vi "Main.vi"(0 "PID On":bool) -> (5 "Total (V)":dbl[](array[slide]) scale=-8.0..8.0, 6 "Force (N)":T3(graph)={"M1 ref force"=20.0, "M2 ref force"=10.768311870905725, "M1 mes force"=3.690819426740976, "M2 mes force"=4.004504201458466})   [LabVIEW 2021]
uses:
  <vilib>/Platform/TimedLoop/XDataNode/timing_clust.ctl
  <vilib>/Platform/TimedLoop/XDataNode/nitl_modes.ctl
  <vilib>/Platform/TimedLoop/XDataNode/wakeup.ctl
  <vilib>/DAQmx/write.llb/DAQmx Write (Digital 1D Bool 1Chan 1Samp).vi
  <vilib>/DAQmx/write.llb/DAQmx Write (Analog 1D DBL NChan 1Samp).vi
  <vilib>/DAQmx/create/channels.llb/DAQmx Create Channel (DO-Digital Output).vi
  <vilib>/DAQmx/create/channels.llb/DAQmx Create Channel (AO-Voltage-Basic).vi
  <vilib>/DAQmx/create/channels.llb/DAQmx Create Channel (AI-Voltage-Basic).vi
  <vilib>/addons/control/pid/pid.llb/PID (DBL).vi
  <vilib>/DAQmx/miscellaneous.llb/DAQmx Fill In Error Info.vi
  <vilib>/Platform/TimedLoop/XDataNode/XDataNode.xnode
  <vilib>/Platform/TimedLoop/XDataNode/XDNodeRunTimeDep.lvlib
  <vilib>/addons/control/pid/NI_PID_pid.lvlib
panel:
  in  "Traj Start":bool
  in  "PID gains":T1={"proportional gain (Kc)"=0.15, "integral time (Ti, min)"=0.0, "derivative time (Td, min)"=0.0} {"derivative time (Td, min)" format="%.3f"; "integral time (Ti, min)" format="%.3f"; "proportional gain (Kc)" format="%.3f"}
  out "output":dbl(slide)=-9.231688129094275 scale=-40.0..40.0
  in  "Numeric":dbl=3.0
  in  "Tab Control":enum32{"PID Gain", "PIN On"}(tab)=enum."PIN On"
  in  "Gains":T2(array[cluster])=[{"proportional gain (Kc)"=0.17, "integral time (Ti, min)"=0.0, "derivative time (Td, min)"=0.0}, {"proportional gain (Kc)"=0.17, "integral time (Ti, min)"=0.0, "derivative time (Td, min)"=0.0}] {"derivative time (Td, min)" format="%.3f"; "integral time (Ti, min)" format="%.3f"; "proportional gain (Kc)" format="%.3f"}
  out "PID (V)":dbl[](array[slide])=[2.7725606974540344, 1.0] scale=-8.0..8.0
  out "Position (mm)":cluster{"Position":dbl, "ref_x (mm)":dbl}(graph)={"Position"=61.544587527295164, "ref_x (mm)"=0.0}
  in  "Loadcell":bool
  in  "Encoder Init":bool
  out "Speed (RPM)":dbl[](array[knob]) scale=-200.0..200.0
  out "time (s)":dbl=637.168
  in  "Set Point":dbl(slide)=19.690402476780186 scale=0.0..40.0
  in  "Motor Enable":bool[](array[boolean])=[FALSE, FALSE]
  in  "stop":bool
  # "FORCE"
  # "TRAJECTORY"
  # "INITIALIZE"
  # "TUNE"
  # "MONITOR"
  # "DEVEL"
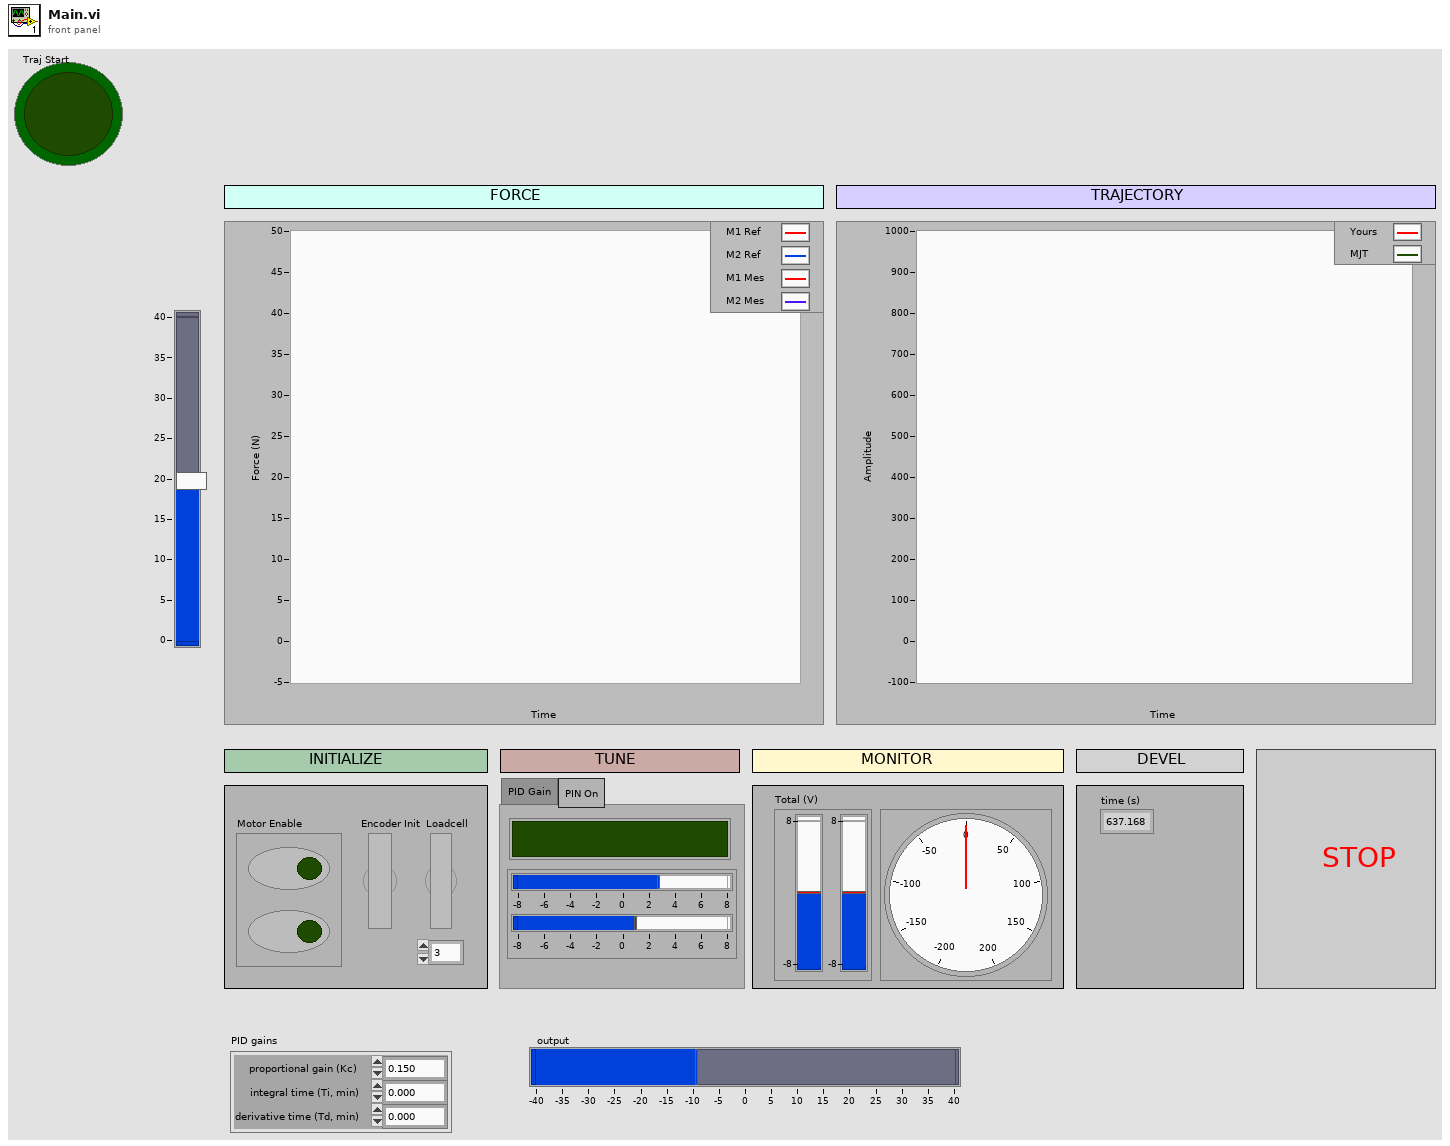
[diagram p1: front panel]
types:
  T1 = cluster{"proportional gain (Kc)":dbl, "integral time (Ti, min)":dbl, "derivative time (Td, min)":dbl}
  T2 = cluster{"proportional gain (Kc)":dbl, "integral time (Ti, min)":dbl, "derivative time (Td, min)":dbl}[]
  T3 = cluster{"M1 ref force":dbl, "M2 ref force":dbl, "M1 mes force":dbl, "M2 mes force":dbl}
  T4 = typedef "XDNodeRunTimeDep.lvlib/timing_clust.ctl" = cluster{"Expected End [f-1]":u64, "Actual End [f-1]":u64, "Finished Late? [f-1]":bool, "Expected End [i-1]":u64, "Actual End [i-1]":u64, "Finished Late? [i-1]":bool, "Expected Start [i]":u64, "Actual Start [i]":u64, "Expected Start [f]":u64, "Actual Start [f]":u64, "Source Name":string, "Structure Name":string, "Period":i64, "Deadline":i64, "Offset":i64, "Start":i64, "Priority":i32, "Timeout":i32, "Mode":T5, "Wakeup Reason":T6, "Error":errorcluster, "Source Type":string, "Secondary Source Type":string, "Global End Time":u64, "Global Start Time":u64, "Frame Duration":u64, "Iteration Duration":u64, "Assigned CPU":i32, "I/O Scan Engine Mode":u32}
  T5 = typedef "XDNodeRunTimeDep.lvlib/nitl_modes.ctl" = enum32{"No Change", "Process missed periods, maintain original phase", "Discard missed periods, maintain original phase", "Process missed periods, ignore original phase", "Discard missed periods, ignore original phase"}
  T6 = typedef "XDNodeRunTimeDep.lvlib/wakeup.ctl" = enum32{"Normal", "Aborted", "Asynchronous wakeup", "Timing source error", "Timed loop error", "Timeout"}
  T7 = cluster{"Total Time":dbl, "Total Length":dbl, "Control Freq":dbl}
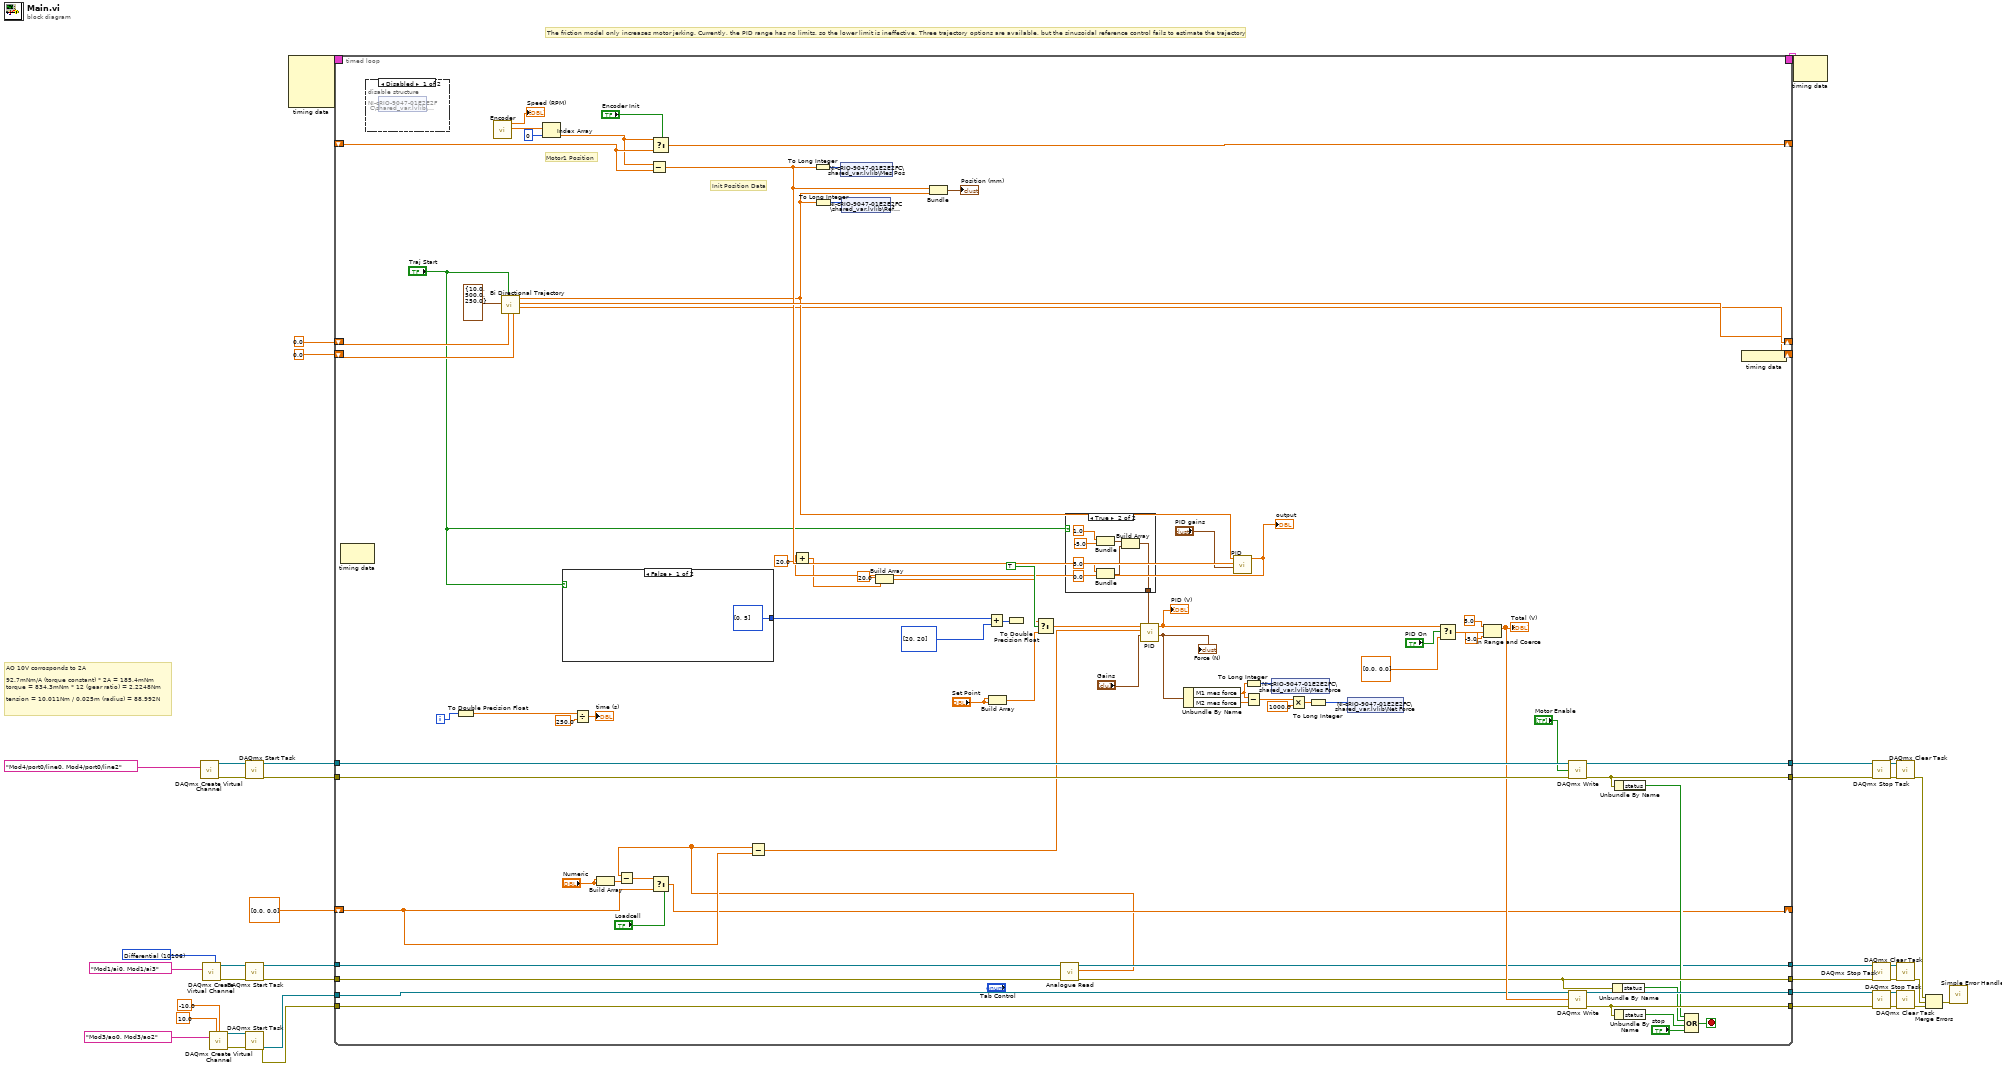
[diagram p0: block diagram]
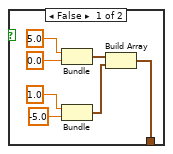
[diagram p3: hidden frame]
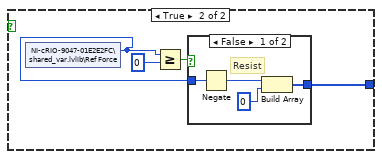
[diagram p4: hidden frame]
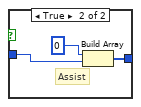
[diagram p5: hidden frame]
diagram:
  w4 = 10106 items=["Default"=-1, "RSE"=10083, "NRSE"=10078, "Differential"=10106, "Pseudodifferential"=12529] ("input terminal configuration")
  # "The friction model only increases motor jerking. Currently, the PID range has no limits, so the lower limit is ineffective. Three trajectory options are available, but the sinusoidal reference control fails to estimate the trajectory"
  # "AO 10V corrosponds to 2A\n\n92.7mNm/A (torque constant) * 2A = 185.4mNm\ntorque = 834.3mNm * 12 (gear ratio) = 2.2248Nm\n\ntension = 10.011Nm / 0.025m (radius) = 88.992N"
  n1 = call-poly <vilib>:"DAQmx Create Virtual Channel.vi"("lines"=tag "Mod4/port0/line0, Mod4/port0/line2") -> ("task out"=w31:refnum<k21>, "error out"=w30:errorcluster)  [unwired: 13 in]
  n2 = call-poly <vilib>:"DAQmx Create Virtual Channel.vi"("input terminal configuration"=w4, "physical channels"=tag "Mod1/ai0, Mod1/ai3") -> ("task out"=w21:refnum<k21>, "error out"=w22:errorcluster)  [unwired: 12 in]
  n3 = call-poly <vilib>:"DAQmx Create Virtual Channel.vi"("maximum value"=10.0 ("AO max"), "minimum value"=-10.0 ("AO min"), "physical channels"=tag "Mod3/ao0, Mod3/ao2" ("Physical Channel(s)")) -> ("task out"=w15:refnum<k21>, "error out"=w14:errorcluster)  [unwired: 11 in]
  n4 = call <vilib>:"DAQmx Start Task.vi"("task/channels in"=w31, "error in"=w30) -> ("task out"=w28:refnum<k21>, "error out"=w27:errorcluster)  [unwired: 12 in]
  n5 = call <vilib>:"DAQmx Start Task.vi"("task/channels in"=w21, "error in"=w22) -> ("task out"=w19:refnum<k21>, "error out"=w18:errorcluster)  [unwired: 12 in]
  n6 = call <vilib>:"DAQmx Start Task.vi"("task/channels in"=w15, "error in"=w14) -> ("task out"=w33:refnum<k21>, "error out"=w32:errorcluster)  [unwired: 12 in]
  n7 = node-c288() -> (w35:T4)  [unwired: 4 in]
  n8 = timed-loop {
    tunnel: [w117] -> w39
    tunnel: [w116] -> w38
    tunnel: [w75] -> w37
    tunnel: [w103] -> w36
    tunnel: w19 -> [w114]
    timing: w35 -> [_]
    timing-out: [_] -> w34
    tunnel: w18 -> [w113]
    tunnel: w33 -> [w74]
    tunnel: w32 -> [w115]
    tunnel: w28 -> [w112]
    tunnel: w27 -> [w111]
    tunnel: [w110] -> w24
    tunnel: [w104] -> w23
    shift-right: [w85] -> _
    shift-left: 0.0 ("total time") -> [w86]
    shift-right: [w80] -> _
    shift-left: _ -> [w78]
    shift-right: [w63] -> _
    shift-left: dbl[] [0.0, 0.0] ("measured force") -> [w64]
    shift-right: [w48] -> _
    shift-left: 0.0 ("total time") -> [w49]
    i -> [w91]
    stop <- w99 stop-if-true
    # "Init Position Data"
    # "Motor1 Position"
    n9 = node-c288() -> ()  [unwired: 1 in, 1 out]
    n10 = disable-structure shown="Disabled" {
      frame Disabled {
        n11 = shared-variable "NI-cRIO-9047-01E2E2FC\\shared_var.lvlib\\Trigger"() -> ()  [unwired: 1 in, 2 out]
      }
      frame Enabled {
      }
    }
    n12 = To Double Precision Float(number=w91) -> (double precision float=w90:dbl)
    n13 = call "Encoder.vi"() -> ("Mes Pos (mm)"=w83:dbl[], "RPM"=→"Speed (RPM)":dbl[])  [unwired: 10 in]
    n14 = call "Bi Directional Trajectory.vi"("Return Time"=w49, "Go Time"=w86, "Traj Start"="Traj Start", "Trajectory Settings"=T7 {"Total Time"=10.0, "Total Length"=500.0, "Control Freq"=250.0}) -> ("Return Next Time"=w48:dbl, "Go Next Time"=w85:dbl, "Output (mm)"=w51:dbl)  [unwired: 5 in]
    n15 = Index Array(array=w83, index=0) -> (element=w42:dbl)
    n16 = case shown="False" "Traj Start" {
      tunnel: [i32[] [0, 5] w138] -> w77
      frame False {
      }
      frame True {
        n17 = shared-variable "NI-cRIO-9047-01E2E2FC\\shared_var.lvlib\\Ref Force"() -> (w137:i32)  [unwired: 1 in, 1 out]
        n18 = Greater Or Equal?(x=w137, y=0) -> (x >= y?=w135:bool)
        n19 = case shown="False" w135 {
          tunnel: w137 -> [w141 w144]
          tunnel: [w142 w145] -> w138
          frame False {
            # "Resist"
            n20 = Negate(x=w141) -> (-x=w139:i32)
            n21 = Build Array(w139, 0 ("element")) -> (w142:i32[])
          }
          frame True {
            # "Assist"
            n22 = Build Array(0 ("element"), w144) -> (w145:i32[])
          }
        }
      }
    }
    n23 = Divide(x=w90, y=250.0) -> (x/y=→"time (s)":dbl)
    n24 = Build Array("Numeric", "Numeric") -> (w53:dbl[])
    n25 = Subtract(x=w42, y=w78) -> (x-y=w52:dbl)
    n26 = Select(t=w42, s="Encoder Init", f=w78) -> (s? t:f=w80:dbl)
    n27 = To Long Integer(number=w52) -> (32bit integer=w58:i32)
    n28 = To Long Integer(number=w51) -> (32bit integer=w59:i32)
    n29 = shared-variable "NI-cRIO-9047-01E2E2FC\\shared_var.lvlib\\Mes Pos"(w58) -> ()  [unwired: 1 in, 1 out]
    n30 = shared-variable "NI-cRIO-9047-01E2E2FC\\shared_var.lvlib\\Ref Pos"(w59) -> ()  [unwired: 1 in, 1 out]
    n31 = Bundle(w52, "Output (mm)"=w51) -> (→"Position (mm)":cluster{dbl, "Output (mm)":dbl})  [unwired: 1 in]
    n32 = Add(x=w77, y=i32[] [20, 20] ("x")) -> (x+y=w73:i32[])
    n33 = Build Array("Set Point", "Set Point") -> (w93:dbl[])
    n34 = To Double Precision Float(number=w73) -> ()  [unwired: 1 out]
    n35 = call "Analogue Read.vi"("error in"=w113, "task/channels in"=w114) -> ("error out"=w103:errorcluster, "measured force"=w61:dbl[], "task out"=w75:refnum<k21>)  [unwired: 6 in, 1 out]
    n36 = Subtract(x=w61, y=w53) -> (x-y=w60:dbl[])
    n37 = Select(t=w60, s="Loadcell", f=w64) -> (s? t:f=w63:dbl[])
    n38 = Subtract(x=w61, y=w64) -> (x-y=w62:dbl[])
    n39 = case shown="True" "Traj Start" {
      tunnel: [w120 w127] -> w66
      frame False {
        n40 = Bundle(5.0, 0.0) -> (w126:cluster{dbl, dbl})  [unwired: 1 in]
        n41 = Bundle(1.0, -5.0) -> (w125:cluster{dbl, dbl})  [unwired: 1 in]
        n42 = Build Array(w126, w125) -> (w120:cluster{dbl, dbl}[])
      }
      frame True {
        n43 = Bundle(1.0, -5.0) -> (w128:cluster{dbl, dbl})  [unwired: 1 in]
        n44 = Bundle(5.0, 0.0) -> (w129:cluster{dbl, dbl})  [unwired: 1 in]
        n45 = Build Array(w128, w129) -> (w127:cluster{dbl, dbl}[])
      }
    }
    n46 = call-poly <vilib>:"PID.vi"("PID gains"="PID gains", "process variable"=w52, "setpoint"=w51) -> ("output"=w45:dbl)  [unwired: 7 in, 1 out]
    "output" <- w45
    n47 = Add(x=w45, y=20.0) -> (x+y=w44:dbl)
    n48 = Build Array(20.0 ("element"), w44) -> (w43:dbl[])
    n49 = Select(t=w43, s=TRUE, f=w93) -> (s? t:f=w70:dbl[])
    n50 = call <vilib>:"PID.vi"("output range"=w66, "PID gains"="Gains", "mes force"=w62, "ref force"=w70) -> ("output cluster"=w55:T3, "PID output"=w97:dbl[])  [unwired: 6 in]
    "Force (N)" <- w55
    "PID (V)" <- w97
    n51 = Unbundle By Name(w55) -> ("M1 mes force"=w67:dbl, "M2 mes force"=w68:dbl)
    n52 = To Long Integer(number=w67) -> (32bit integer=w69:i32)
    n53 = Subtract(x=w67, y=w68) -> (x-y=w72:dbl)
    n54 = shared-variable "NI-cRIO-9047-01E2E2FC\\shared_var.lvlib\\Mes Force"(w69) -> ()  [unwired: 1 in, 1 out]
    n55 = Multiply(x=w72, y=1000.0) -> (x*y=w56:dbl)
    n56 = To Long Integer(number=w56) -> (32bit integer=w57:i32)
    n57 = shared-variable "NI-cRIO-9047-01E2E2FC\\shared_var.lvlib\\Net Force"(w57) -> ()  [unwired: 1 in, 1 out]
    n58 = Select(t=w97, s="PID On", f=dbl[] [0.0, 0.0]) -> (s? t:f=w95:dbl[])
    n59 = In Range and Coerce(upper limit=5.0, x=w95, lower limit=-5.0) -> (coerced(x)=w105:dbl[])  [unwired: 1 out]
    "Total (V)" <- w105
    n60 = call-poly <vilib>:"DAQmx Write.vi"("task/channels in"=w112, "data"="Motor Enable", "error in"=w111) -> ("task out"=w110:refnum<k21>, "error out"=w104:errorcluster)  [unwired: 10 in, 1 out]
    n61 = call-poly <vilib>:"DAQmx Write.vi"("task/channels in"=w74, "data"=w105, "error in"=w115) -> ("task out"=w117:refnum<k21>, "error out"=w116:errorcluster)  [unwired: 10 in, 1 out]
    n62 = Unbundle By Name(w103) -> ("status"=w101:bool)
    n63 = Unbundle By Name(w104) -> ("status"=w100:bool)
    n64 = Unbundle By Name(w116) -> ("status"=w102:bool)
    n65 = Compound Arithmetic op=OR(w100, w101, w102, "stop") -> (w99:bool)
    n66 = node-c288() -> ()  [unwired: 1 out]
  }
  n67 = node-c288(w34) -> ()  [unwired: 1 out]
  n68 = call <vilib>:"DAQmx Stop Task.vi"("task/channels in"=w24, "error in"=w23) -> ("task out"=w26:refnum<k21>, "error out"=w25:errorcluster)  [unwired: 12 in]
  n69 = call <vilib>:"DAQmx Stop Task.vi"("task/channels in"=w37, "error in"=w36) -> ("task out"=w10:refnum<k21>, "error out"=w9:errorcluster)  [unwired: 12 in]
  n70 = call <vilib>:"DAQmx Stop Task.vi"("task/channels in"=w39, "error in"=w38) -> ("task out"=w12:refnum<k21>, "error out"=w11:errorcluster)  [unwired: 12 in]
  n71 = call <vilib>:"DAQmx Clear Task.vi"("task in"=w26, "error in"=w25) -> ("error out"=w5:errorcluster)  [unwired: 13 in]
  n72 = call <vilib>:"DAQmx Clear Task.vi"("task in"=w10, "error in"=w9) -> ("error out"=w6:errorcluster)  [unwired: 13 in]
  n73 = call <vilib>:"DAQmx Clear Task.vi"("task in"=w12, "error in"=w11) -> ("error out"=w7:errorcluster)  [unwired: 13 in]
  n74 = Merge Errors(w5, w6, w7) -> (w8:errorcluster)
  n75 = call <vilib>:"Simple Error Handler.vi"("error in (no error)"=w8) -> ()  [unwired: 4 in, 5 out]
